vi "OFBS_savePaths.vi"(8 "error in (no error)":errorcluster, 10 "Paths":T1, 11 "BandGlobalOpt in":refnum<class "OptFreqBandsSearch.lvclass">) -> (0 "error out":errorcluster, 3 "BandGlobalOpt out":refnum<class "OptFreqBandsSearch.lvclass">)   [LabVIEW 2016, in "Optimal Frequency Bands Search.lvlib" / "OptFreqBandsSearch.lvclass"]
doc: "Метод, реализующий сохранение путей к файлам в приватных данных класса"
uses:
  OptFreqBandsSearch.lvclass
  OptFreqBandsSearch.lvclass/OptFreqBandsSearch.ctl
panel:
  # "This VI is a part of BCI Design library, http://www.ru-bci.org \nCopyright © 2020, Sotnikov Peter, All rights reserved. License: CC BY-NC 4.0"
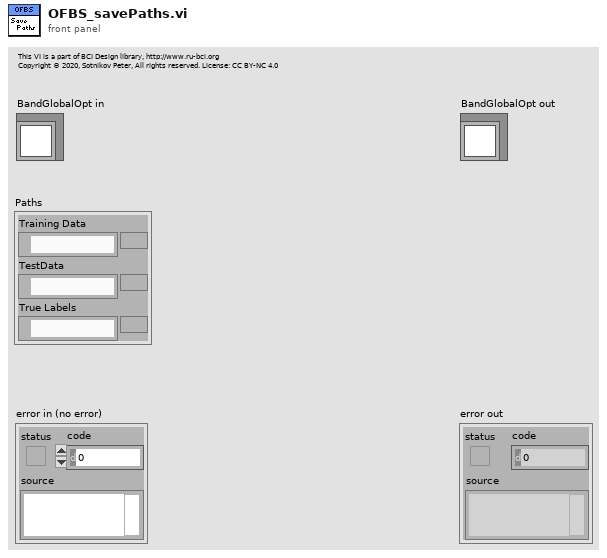
[diagram p1: front panel]
types:
  T1 = cluster{"Training Data":path, "TestData":path, "True Labels":path}
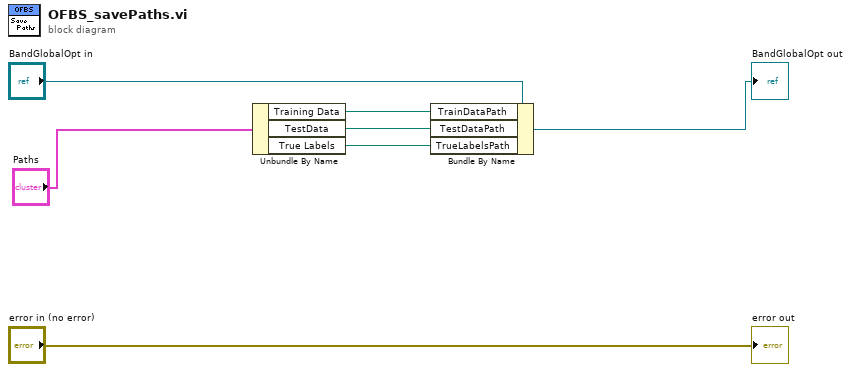
[diagram p0: block diagram]
diagram:
  n1 = Unbundle By Name("Paths") -> ("Training Data"=w3:path, "TestData"=w2:path, "True Labels"=w1:path)
  n2 = Bundle By Name(cluster="BandGlobalOpt in", "TrainDataPath"=w3, "TestDataPath"=w2, "TrueLabelsPath"=w1) -> (→"BandGlobalOpt out":refnum<class "OptFreqBandsSearch.lvclass">)
  "error out" <- "error in (no error)"
